vi "Img_Draw_Point.vi"(4 "Color":u32(colorbox)=16711680, 6 "diameter":u16=10, 8 "error in (no error)":errorcluster, 10 "Point Coordinates":cluster{"X":dbl, "Y":dbl}, 11 "Image In":T1) -> (0 "error out":errorcluster, 3 "Image Out":T1)   [LabVIEW 2021, in "Framework_lib.lvlib"]
uses:
  QMH/Framework_lib.lvlib
  <vilib>/vision/Image Controls.llb/IMAQ Image.ctl
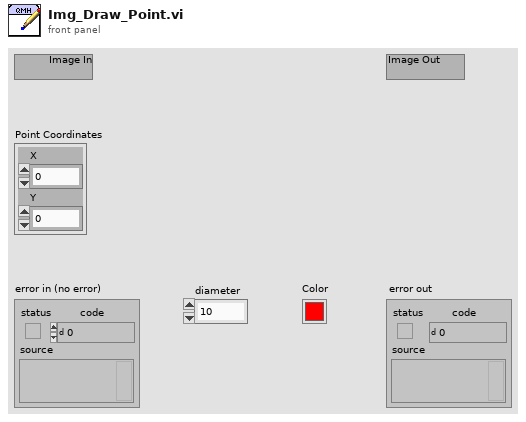
[diagram p1: front panel]
types:
  T1 = typedef "IMAQ Image.ctl" = refnum<image>
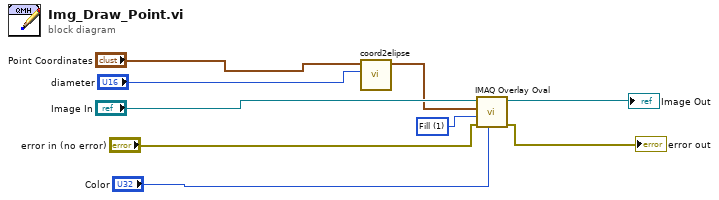
[diagram p0: block diagram]
diagram:
  w2 = u32 1 items=["Frame", "Fill"] ("Drawing Mode (Frame)")
  n1 = call "coord2elipse.vi"("diameter"="diameter", "Point Coordinates"="Point Coordinates") -> ("Cluster"=w1:cluster{dbl, dbl, dbl, dbl})  [unwired: 9 in]
  n2 = call "IMAQ Overlay Oval"("Color"="Color", "error in (no error)"="error in (no error)", "Drawing Mode (Frame)"=w2, "Bounding Rectangle"=w1, "Image"="Image In") -> ("error out"=→"error out":errorcluster, "Image Out"=→"Image Out":T1)  [unwired: 5 in]
